vi "Parallelism-LocalVariable.vi"() -> ()   [LabVIEW 2020]
doc: "Use this template to build a master/slave design pattern. The master loop always executes. It notifies one or more slave loops to execute their code. The slave loop(s) continue executing until they complete, then wait for another notification. Contrast this with the Producer/Consumer pattern in which the consumer loops execute only when they have data in their queue."
panel:
  out "error out":errorcluster
  in  "error in":errorcluster
  in  "stop":bool
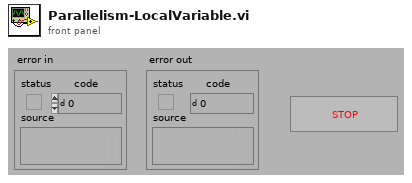
[diagram p1: front panel]
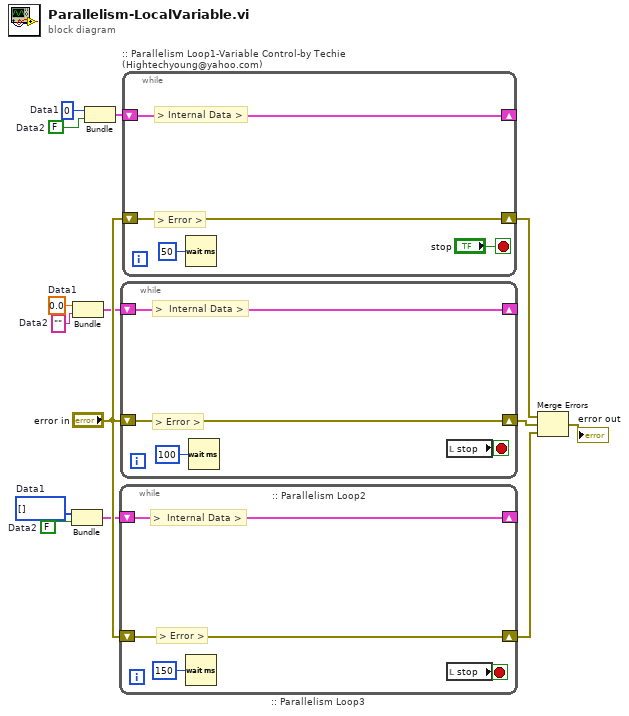
[diagram p0: block diagram]
diagram:
  w1 = i32[] []  # Data1
  w2 = ""  # Data2
  w4 = FALSE  # Data2
  w7 = 0.0  # Data1
  w8 = FALSE  # Data2
  w9 = 0  # Data1
  n1 = Bundle("Data1"=w1, "Data2"=w4) -> (w3:cluster{"Data1":i32[], "Data2":bool})  [unwired: 1 in]
  n2 = Bundle("Data1"=w7, "Data2"=w2) -> (w6:cluster{"Data1":dbl, "Data2":string})  [unwired: 1 in]
  n3 = Bundle("Data1"=w9, "Data2"=w8) -> (w5:cluster{"Data1":i32, "Data2":bool})  [unwired: 1 in]
  n4 = while ":: Parallelism Loop3" {
    shift-right: [w16] -> w10
    shift-left: "error in" -> [w16]
    shift-right: [w17] -> _
    shift-left: w3 -> [w17]
    stop <- w15 stop-if-true
    # "> Error >"
    # ">  Internal Data >"
    n5 = Wait (ms)(milliseconds to wait=u32 150) -> ()  [unwired: 1 out]
    n6 = local read "stop"() -> (w15:bool)
  }
  n7 = while ":: Parallelism Loop2" {
    shift-right: [w20] -> w12
    shift-left: "error in" -> [w20]
    shift-right: [w22] -> _
    shift-left: w6 -> [w22]
    stop <- w19 stop-if-true
    # "> Error >"
    # ">  Internal Data >"
    n8 = Wait (ms)(milliseconds to wait=u32 100) -> ()  [unwired: 1 out]
    n9 = local read "stop"() -> (w19:bool)
  }
  n10 = while ":: Parallelism Loop1-Variable Control-by Techie (Hightechyoung@yahoo.com)" {
    shift-right: [w24] -> w11
    shift-left: "error in" -> [w24]
    shift-right: [w26] -> _
    shift-left: w5 -> [w26]
    stop <- "stop" stop-if-true
    # "> Error >"
    # "> Internal Data >"
    n11 = Wait (ms)(milliseconds to wait=u32 50) -> ()  [unwired: 1 out]
  }
  n12 = Merge Errors(w11, w12, w10) -> (→"error out":errorcluster)
